vi "TestPcTcpSample.vi"() -> ()   [LabVIEW 2021]
doc: "ホール測定PC用TCP通信サンプル"
uses:
  SubVI/HallMeasurementStatus.ctl
  SubVI/TcpCommunicationClientCMD.ctl
panel:
  out "EstimatedRefractiveIndex":dbl
  out "EstimatedThickness[nm]":dbl
  out "Temperature[degC]":dbl
  out "TcpOK?":bool
  in  "Start":bool
  in  "DataFilePath":path=path "Test"
  out "SampleName":string
  in  "Status":T1
  out "ReadData":string
  in  "Send Data":string
  in  "Send":bool
  in  "ポート":u16=8501
  in  "中央PCアドレス":string="localhost"
  in  "停止":bool
  # "テストPC用TCP通信サンプル"
  # "1. マネージャーPC用TCP通信サンプル（ManagerTcpSample.exe）を実行します。\n\n2. テスト測定PC用TCP通信サンプル（TestTcpSample.exe）を実行します。\n　ManagerTcpSample.exeのリモートアドレスに、こちらのIPアドレスが表示されます。\n\n3. ManagerTcpSample.exeのエリプソ測定PCアドレスにアドレスを入力します。\n\n4. ManagerTcpSample.exeのボタンを押すと対応するコマンドが送られます。\n\n5. 受信したコマンドに応じて自動で返信を送信します。\n\n6. コマンドに対応してStatusやFilePath、StartやOKのLEDが変化します。\n\n7. 停止時はこちらのソフトを先に止めます。"
  # "↑Startが点灯中はStatusコマンドに\n応答しない。クリックして解除します。"
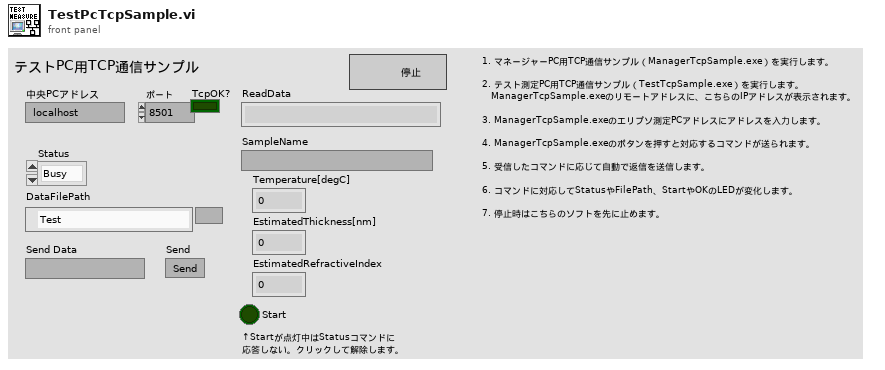
[diagram p1: front panel]
types:
  T1 = typedef "HallMeasurementStatus.ctl" = enum16{"Busy", "Ready", "Done", "Error"}
  T2 = typedef "TcpCommunicationClientCMD.ctl" = enum16{"Read", "Write", "Close"}
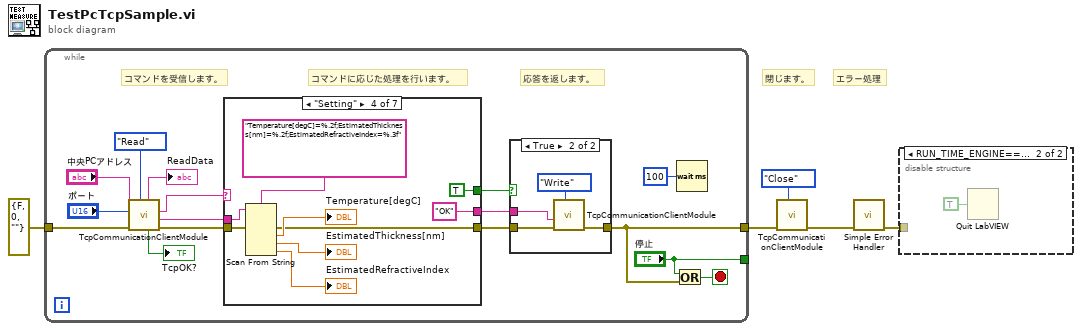
[diagram p0: block diagram]
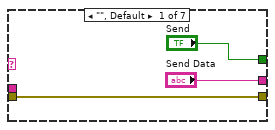
[diagram p4: hidden frame]
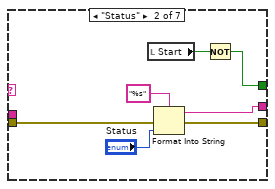
[diagram p5: hidden frame]
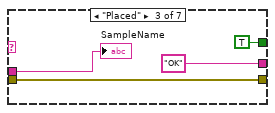
[diagram p6: hidden frame]
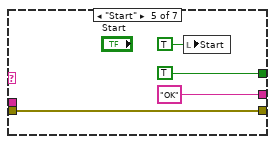
[diagram p7: hidden frame]
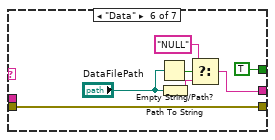
[diagram p8: hidden frame]
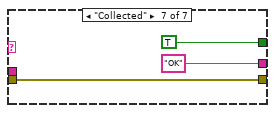
[diagram p9: hidden frame]
diagram:
  # "エラー処理"
  # "閉じます。"
  n1 = while {
    tunnel: ["停止"] -> _
    tunnel: [w10] -> w3
    tunnel: errorcluster {"status"=FALSE, "code"=0, "source"=""} ("エラー入力（エラーなし）") -> [w17]
    stop <- w21 stop-if-true
    # "応答を返します。"
    # "コマンドに応じた処理を行います。"
    # "コマンドを受信します。"
    n2 = call "TcpCommunicationClientModule.vi"("TcpCommunicationClientCMD"=TcpCommunicationClientCMD."Read", "エラー入力（エラーなし）"=w17, "ポート"="ポート", "アドレス"="中央PCアドレス") -> ("エラー出力"=w19:errorcluster, "Data"=w7:string, "Command"=w8:string, "TcpOK?"=→"TcpOK?":bool, "ReadData"=→"ReadData":string)  [unwired: 3 in]
    n3 = case shown="\"Setting\"" w8 {
      tunnel: w7 -> [_ _ w37 w47 _ _ _]
      tunnel: ["Send Data" w35 "OK" ("Send Data") "OK" ("Send Data") "OK" ("Send Data") w55 "OK" ("Send Data")] -> w12
      tunnel: ["Send" w30 TRUE ("Send") TRUE ("Send") TRUE ("Send") TRUE ("Send") TRUE ("Send")] -> w13
      tunnel: w19 -> [w27 w33 w39 w43 w52 w59 w62]
      tunnel: [w27 w32 w39 w42 w52 w59 w62] -> w11
      frame "", Default {
      }
      frame "Status" {
        n4 = local read "Start"() -> (w31:bool)
        n5 = Format Into String(format string="%s" ("形式文字列"), error in=w33, "Status") -> (resulting string=w35:string, error out=w32:errorcluster)  [unwired: 1 in]
        n6 = Not(x=w31) -> (.not. x?=w30:bool)
      }
      frame "Placed" {
        "SampleName" <- w37
      }
      frame "Setting" {
        n7 = Scan From String(format string="Temperature[degC]=%.2f;EstimatedThickness[nm]=%.2f;EstimatedRefractiveIndex=%.3f", input string=w47, error in=w43) -> (error out=w42:errorcluster, output 1=→"Temperature[degC]":dbl, output 2=→"EstimatedThickness[nm]":dbl, output 3=→"EstimatedRefractiveIndex":dbl)  [unwired: 4 in, 2 out]
      }
      frame "Start" {
        n8 = local write "Start"(TRUE) -> ()
      }
      frame "Data" {
        n9 = Empty String/Path?(string/path="DataFilePath") -> (empty?=w57:bool)
        n10 = Path To String(path="DataFilePath") -> (string=w56:string)
        n11 = Select(t="NULL", s=w57, f=w56) -> (s? t:f=w55:string)
      }
      frame "Collected" {
      }
    }
    n12 = case shown="True" w13 {
      tunnel: w11 -> [w22 w26]
      tunnel: [w22 w25] -> w10
      tunnel: w12 -> [_ w23]
      frame False {
      }
      frame True {
        n13 = call "TcpCommunicationClientModule.vi"("TcpCommunicationClientCMD"=TcpCommunicationClientCMD."Write", "エラー入力（エラーなし）"=w26, "WriteData"=w23) -> ("エラー出力"=w25:errorcluster)  [unwired: 4 in, 4 out]
      }
    }
    n14 = Or(x="停止", y=w10) -> (x .or. y?=w21:bool)
    n15 = Wait (ms)(milliseconds to wait=u32 100 ("ミリ秒待機時間")) -> ()  [unwired: 1 out]
  }
  n16 = call "TcpCommunicationClientModule.vi"("TcpCommunicationClientCMD"=TcpCommunicationClientCMD."Close", "エラー入力（エラーなし）"=w3) -> ("エラー出力"=w2:errorcluster)  [unwired: 5 in, 4 out]
  n17 = call <vilib>:"Simple Error Handler.vi"("error in (no error)"=w2) -> ("error out"=w1:errorcluster)  [unwired: 1 in, 7 out]
  n18 = disable-structure shown="RUN_TIME_ENGINE==True" {
    disable-tunnel: w1 -> [_ _]
    frame condition #0 (active) {
    }
    frame condition #1 {
      n19 = Quit LabVIEW(quit? (T)=TRUE) -> ()
    }
  }
